vi "test-Mecanum-Odometry-Test1.vi"() -> (3 "All tests passed":bool)   [LabVIEW 2019]
uses:
  <vilib>/Rock Robotics/WPI/ThirdParty/JAS_Junk/TrajLib/Trajectory_Library.lvlib
panel:
  out "Test 4":bool
  out "Test 3":bool
  out "Test 2":bool
  out "Test 1":bool
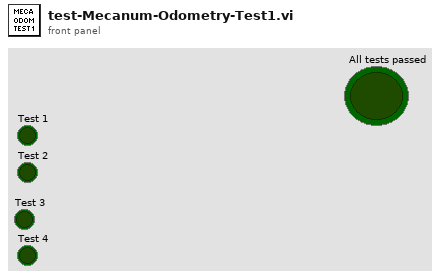
[diagram p1: front panel]
types:
  T1 = typedef "Trajectory_Library.lvlib/ROTATION2D.ctl" = cluster{"VALUE":dbl, "COS":dbl, "SIN":dbl}
  T2 = typedef "Trajectory_Library.lvlib/POSE2D.ctl" = cluster{"TRANSLATION":T3, "ROTATION":T1}
  T3 = typedef "Trajectory_Library.lvlib/TRANSLATION2D.ctl" = cluster{"X":dbl, "Y":dbl}
  T4 = typedef "Trajectory_Library.lvlib/MECA_WHEEL_SPEEDS.ctl" = cluster{"FrontLeftSpeed":dbl, "FrontRightSpeed":dbl, "RearLeftSpeed":dbl, "RearRightSpeed":dbl}
  T5 = typedef "Trajectory_Library.lvlib/MECA_DRIVE_KINEMATICS.ctl" = cluster{"FrontLeft":T3, "FrontRight":T3, "RearLeft":T3, "RearRight":T3, "InverseKinematics":T6, "ForwardKinematics":T6, "PrevCoR":T3}
  T6 = typedef "NI_Matrix.lvlib/RealMatrix.ctl" = dbl[][]
  T7 = typedef "Trajectory_Library.lvlib/MECA_DRIVE_ODOMETRY.ctl" = cluster{"POSE":T2, "PrevTime":dbl, "GyroOffset":T1, "PreviousAngle":T1, "Kinematics":T5}
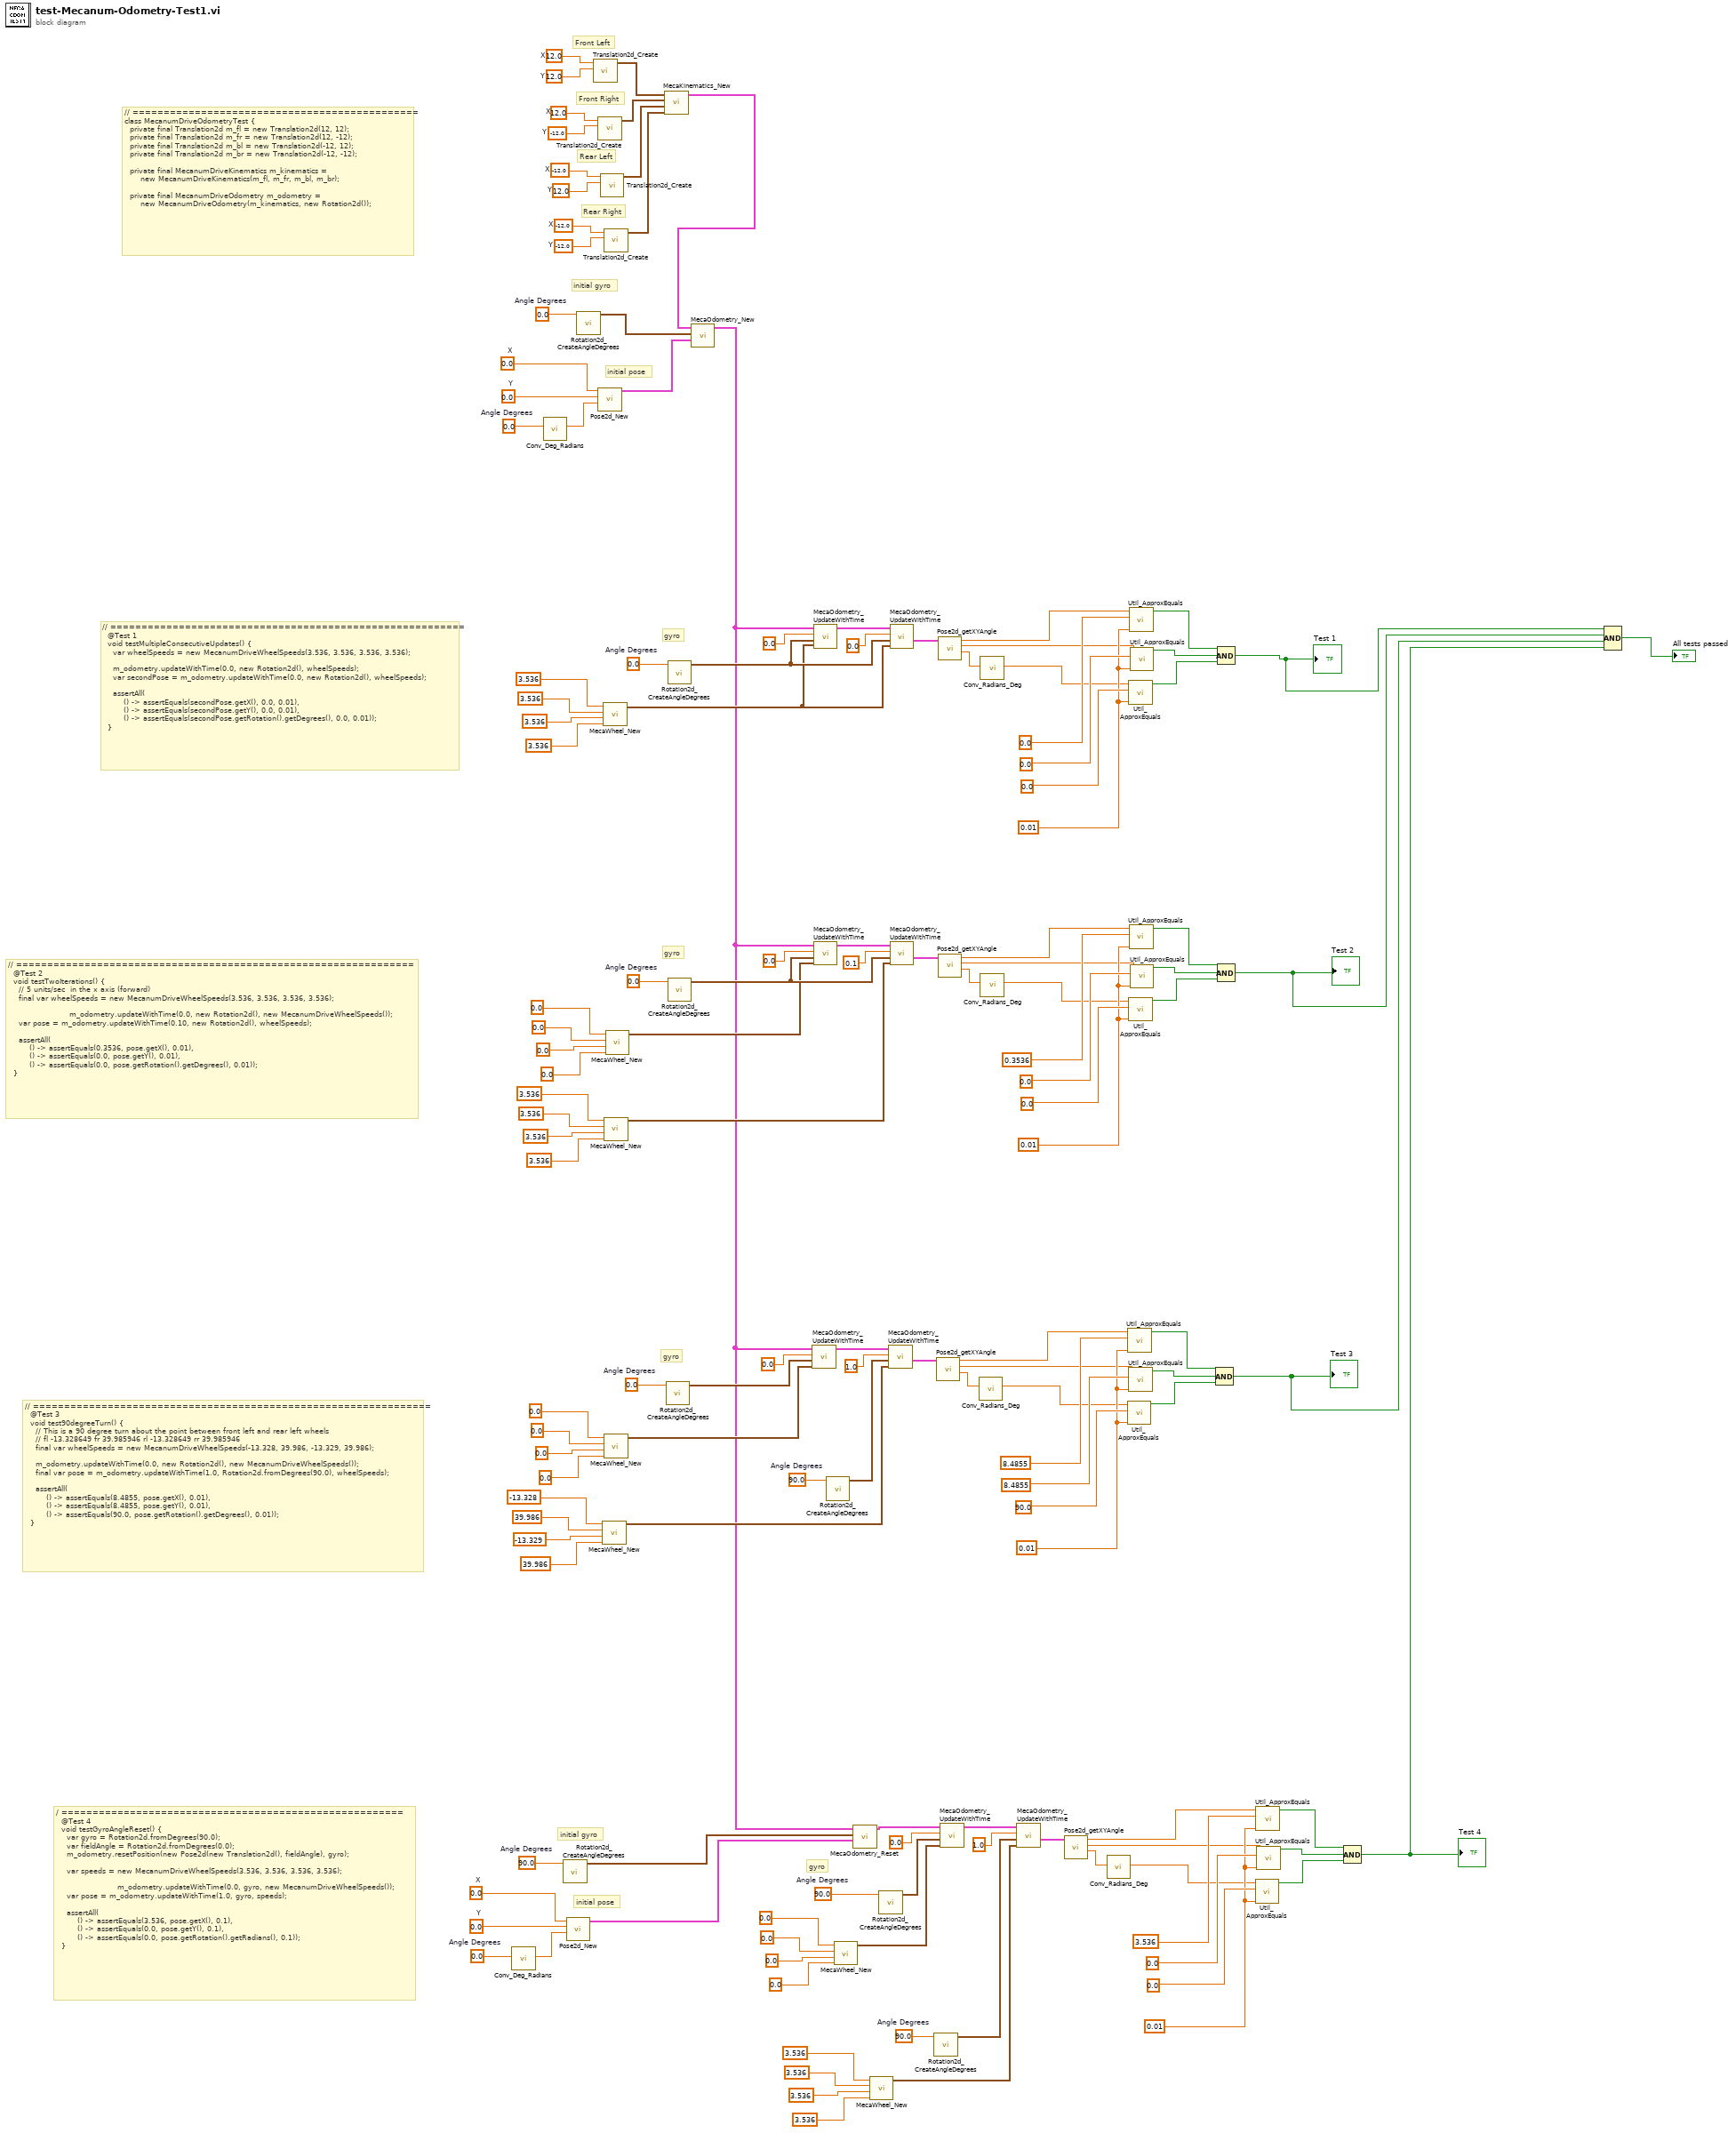
[diagram p0: block diagram]
diagram:
  w6 = 90.0  # Angle Degrees
  w10 = 0.0  # X
  w9 = 0.0  # Y
  w7 = 0.0  # Angle Degrees
  w14 = 90.0  # Angle Degrees
  w28 = 90.0  # Angle Degrees
  w35 = 0.01 ("Tolerance")
  w44 = 90.0  # Angle Degrees
  w58 = 0.0  # Angle Degrees
  w65 = 0.01 ("Tolerance")
  w86 = 0.0  # Angle Degrees
  w93 = 0.01 ("Tolerance")
  w108 = 0.0  # Angle Degrees
  w115 = 0.0  # Angle Degrees
  w120 = 0.0  # X
  w119 = 0.0  # Y
  w117 = 0.0  # Angle Degrees
  w121 = 0.01 ("Tolerance")
  w136 = -12.0  # X
  w135 = -12.0  # Y
  w134 = -12.0  # X
  w133 = 12.0  # Y
  w132 = 12.0  # X
  w131 = -12.0  # Y
  w130 = 12.0  # X
  w129 = 12.0  # Y
  # "initial gyro"
  # "initial pose"
  # "gyro"
  # "/ =======================================================\n  @Test 4\n  void testGyroAngleReset() {\n    var gyro = Rotation2d.fromDegrees(90.0);\n    var fieldAngle = Rotation2d.fromDegrees(0.0);\n    m_odometry.resetPosition(new Pose2d(new Translation2d(), fieldAngle), gyro);\n\n    var speeds = new MecanumDriveWheelSpeeds(3.536, 3.536, 3.536, 3.536);\n\n                       m_odometry.updateWithTime(0.0, gyro, new MecanumDriveWheelSpeeds());\n    var pose = m_odometry.updateWithTime(1.0, gyro, speeds);\n\n    assertAll(\n        () -> assertEquals(3.536, pose.getX(), 0.1),\n        () -> assertEquals(0.0, pose.getY(), 0.1),\n        () -> assertEquals(0.0, pose.getRotation().getRadians(), 0.1));\n  }"
  # "gyro"
  # "// ================================================================\n  @Test 3\n  void test90degreeTurn() {\n    // This is a 90 degree turn about the point between front left and rear left wheels\n    // fl -13.328649 fr 39.985946 rl -13.328649 rr 39.985946\n    final var wheelSpeeds = new MecanumDriveWheelSpeeds(-13.328, 39.986, -13.329, 39.986);\n\n    m_odometry.updateWithTime(0.0, new Rotation2d(), new MecanumDriveWheelSpeeds());\n    final var pose = m_odometry.updateWithTime(1.0, Rotation2d.fromDegrees(90.0), wheelSpeeds);\n\n    assertAll(\n        () -> assertEquals(8.4855, pose.getX(), 0.01),\n        () -> assertEquals(8.4855, pose.getY(), 0.01),\n        () -> assertEquals(90.0, pose.getRotation().getDegrees(), 0.01));\n  }"
  # "gyro"
  # "// ================================================================\n  @Test 2\n  void testTwoIterations() {\n    // 5 units/sec  in the x axis (forward)\n    final var wheelSpeeds = new MecanumDriveWheelSpeeds(3.536, 3.536, 3.536, 3.536);\n\n                       m_odometry.updateWithTime(0.0, new Rotation2d(), new MecanumDriveWheelSpeeds());\n    var pose = m_odometry.updateWithTime(0.10, new Rotation2d(), wheelSpeeds);\n\n    assertAll(\n        () -> assertEquals(0.3536, pose.getX(), 0.01),\n        () -> assertEquals(0.0, pose.getY(), 0.01),\n        () -> assertEquals(0.0, pose.getRotation().getDegrees(), 0.01));\n  }"
  # "gyro"
  # "initial gyro"
  # "initial pose"
  # "// =========================================================\n  @Test 1\n  void testMultipleConsecutiveUpdates() {\n    var wheelSpeeds = new MecanumDriveWheelSpeeds(3.536, 3.536, 3.536, 3.536);\n\n    m_odometry.updateWithTime(0.0, new Rotation2d(), wheelSpeeds);\n    var secondPose = m_odometry.updateWithTime(0.0, new Rotation2d(), wheelSpeeds);\n\n    assertAll(\n        () -> assertEquals(secondPose.getX(), 0.0, 0.01),\n        () -> assertEquals(secondPose.getY(), 0.0, 0.01),\n        () -> assertEquals(secondPose.getRotation().getDegrees(), 0.0, 0.01));\n  }"
  # "Rear Right"
  # "Rear Left"
  # "Front Right"
  # "Front Left"
  # "// ==============================================\nclass MecanumDriveOdometryTest {\n  private final Translation2d m_fl = new Translation2d(12, 12);\n  private final Translation2d m_fr = new Translation2d(12, -12);\n  private final Translation2d m_bl = new Translation2d(-12, 12);\n  private final Translation2d m_br = new Translation2d(-12, -12);\n\n  private final MecanumDriveKinematics m_kinematics =\n      new MecanumDriveKinematics(m_fl, m_fr, m_bl, m_br);\n\n  private final MecanumDriveOdometry m_odometry =\n      new MecanumDriveOdometry(m_kinematics, new Rotation2d());"
  n1 = call <vilib>:"Conv_Deg_Radians.vi"("Degress"=w7) -> ("Radians"=w8:dbl)  [unwired: 10 in]
  n2 = call <vilib>:"Conv_Deg_Radians.vi"("Degress"=w117) -> ("Radians"=w118:dbl)  [unwired: 10 in]
  n3 = call <vilib>:"Rotation2d_CreateAngleDegrees.vi"("Angle_Degrees"=w6) -> ("ROTATION"=w5:T1)  [unwired: 10 in]
  n4 = call <vilib>:"Pose2d_New.vi"("Heading"=w8, "Y"=w9, "X"=w10) -> ("out POSe"=w4:T2)  [unwired: 8 in]
  n5 = call <vilib>:"Rotation2d_CreateAngleDegrees.vi"("Angle_Degrees"=w115) -> ("ROTATION"=w2:T1)  [unwired: 10 in]
  n6 = call <vilib>:"Translation2d_Create.vi"("Y"=w129, "X"=w130) -> ("TRANSLATION"=w137:T3)  [unwired: 9 in]
  n7 = call <vilib>:"Translation2d_Create.vi"("Y"=w131, "X"=w132) -> ("TRANSLATION"=w138:T3)  [unwired: 9 in]
  n8 = call <vilib>:"Pose2d_New.vi"("Heading"=w118, "Y"=w119, "X"=w120) -> ("out POSe"=w116:T2)  [unwired: 8 in]
  n9 = call <vilib>:"Translation2d_Create.vi"("Y"=w133, "X"=w134) -> ("TRANSLATION"=w139:T3)  [unwired: 9 in]
  n10 = call <vilib>:"MecaWheel_New.vi"("RearRightSpeed"=39.986, "RearLeftSpeed"=-13.329, "FrontRightSpeed"=39.986, "FrontLeftSpeed"=-13.328) -> ("MECA_WHEEL_SPEEDS"=w50:T4)  [unwired: 7 in]
  n11 = call <vilib>:"MecaWheel_New.vi"("RearRightSpeed"=3.536, "RearLeftSpeed"=3.536, "FrontRightSpeed"=3.536, "FrontLeftSpeed"=3.536) -> ("MECA_WHEEL_SPEEDS"=w100:T4)  [unwired: 7 in]
  n12 = call <vilib>:"Translation2d_Create.vi"("Y"=w135, "X"=w136) -> ("TRANSLATION"=w140:T3)  [unwired: 9 in]
  n13 = call <vilib>:"MecaWheel_New.vi"("RearRightSpeed"=3.536, "RearLeftSpeed"=3.536, "FrontRightSpeed"=3.536, "FrontLeftSpeed"=3.536) -> ("MECA_WHEEL_SPEEDS"=w78:T4)  [unwired: 7 in]
  n14 = call <vilib>:"MecaWheel_New.vi"("RearRightSpeed"=0.0, "RearLeftSpeed"=0.0, "FrontRightSpeed"=0.0, "FrontLeftSpeed"=0.0) -> ("MECA_WHEEL_SPEEDS"=w45:T4)  [unwired: 7 in]
  n15 = call <vilib>:"MecaWheel_New.vi"("RearRightSpeed"=0.0, "RearLeftSpeed"=0.0, "FrontRightSpeed"=0.0, "FrontLeftSpeed"=0.0) -> ("MECA_WHEEL_SPEEDS"=w73:T4)  [unwired: 7 in]
  n16 = call <vilib>:"MecaKinematics_New.vi"("RearRight"=w140, "RearLeft"=w139, "FrontRight"=w138, "FrontLeft"=w137) -> ("MECA_DRIVE_KINEMATICS"=w1:T5)  [unwired: 7 in]
  n17 = call <vilib>:"Rotation2d_CreateAngleDegrees.vi"("Angle_Degrees"=w58) -> ("ROTATION"=w56:T1)  [unwired: 10 in]
  n18 = call <vilib>:"Rotation2d_CreateAngleDegrees.vi"("Angle_Degrees"=w108) -> ("ROTATION"=w106:T1)  [unwired: 10 in]
  n19 = call <vilib>:"Rotation2d_CreateAngleDegrees.vi"("Angle_Degrees"=w86) -> ("ROTATION"=w84:T1)  [unwired: 10 in]
  n20 = call <vilib>:"MecaOdometry_New.vi"("Initial Pose2d"=w116, "GyroOffset"=w2, "Mecanum Kinematics"=w1) -> ("MECA_DRIVE_ODOMETRY"=w11:T7)  [unwired: 8 in]
  n21 = call <vilib>:"MecaOdometry_UpdateWithTime.vi"("WheelSpeeds"=w45, "GyroAngle"=w56, "CurrentTime"=0.0, "in MECA_DRIVE_ODOMETRY"=w11) -> ("out MECA_DRIVE_ODOMETRY"=w60:T7)  [unwired: 6 in, 1 out]
  n22 = call <vilib>:"MecaOdometry_UpdateWithTime.vi"("WheelSpeeds"=w100, "GyroAngle"=w106, "CurrentTime"=0.0, "in MECA_DRIVE_ODOMETRY"=w11) -> ("out MECA_DRIVE_ODOMETRY"=w110:T7)  [unwired: 6 in, 1 out]
  n23 = call <vilib>:"MecaOdometry_UpdateWithTime.vi"("WheelSpeeds"=w73, "GyroAngle"=w84, "CurrentTime"=0.0, "in MECA_DRIVE_ODOMETRY"=w11) -> ("out MECA_DRIVE_ODOMETRY"=w88:T7)  [unwired: 6 in, 1 out]
  n24 = call <vilib>:"Rotation2d_CreateAngleDegrees.vi"("Angle_Degrees"=w44) -> ("ROTATION"=w43:T1)  [unwired: 10 in]
  n25 = call <vilib>:"MecaWheel_New.vi"("RearRightSpeed"=0.0, "RearLeftSpeed"=0.0, "FrontRightSpeed"=0.0, "FrontLeftSpeed"=0.0) -> ("MECA_WHEEL_SPEEDS"=w15:T4)  [unwired: 7 in]
  n26 = call <vilib>:"MecaOdometry_Reset.vi"("POSE"=w4, "GyroOffset"=w5, "in MECA_DRIVE_ODOMETRY"=w11) -> ("out MECA_DRIVE_ODOMETRY"=w12:T7)  [unwired: 8 in]
  n27 = call <vilib>:"MecaWheel_New.vi"("RearRightSpeed"=3.536, "RearLeftSpeed"=3.536, "FrontRightSpeed"=3.536, "FrontLeftSpeed"=3.536) -> ("MECA_WHEEL_SPEEDS"=w20:T4)  [unwired: 7 in]
  n28 = call <vilib>:"Rotation2d_CreateAngleDegrees.vi"("Angle_Degrees"=w28) -> ("ROTATION"=w26:T1)  [unwired: 10 in]
  n29 = call <vilib>:"MecaOdometry_UpdateWithTime.vi"("WheelSpeeds"=w50, "GyroAngle"=w43, "CurrentTime"=1.0, "in MECA_DRIVE_ODOMETRY"=w60) -> ("POSE"=w55:T2)  [unwired: 6 in, 1 out]
  n30 = call <vilib>:"MecaOdometry_UpdateWithTime.vi"("WheelSpeeds"=w100, "GyroAngle"=w106, "CurrentTime"=0.0, "in MECA_DRIVE_ODOMETRY"=w110) -> ("POSE"=w105:T2)  [unwired: 6 in, 1 out]
  n31 = call <vilib>:"MecaOdometry_UpdateWithTime.vi"("WheelSpeeds"=w78, "GyroAngle"=w84, "CurrentTime"=0.1, "in MECA_DRIVE_ODOMETRY"=w88) -> ("POSE"=w83:T2)  [unwired: 6 in, 1 out]
  n32 = call <vilib>:"Rotation2d_CreateAngleDegrees.vi"("Angle_Degrees"=w14) -> ("ROTATION"=w13:T1)  [unwired: 10 in]
  n33 = call <vilib>:"Pose2d_getXYAngle.vi"("in POSE"=w55) -> ("Angle"=w54:dbl, "Y"=w52:dbl, "X"=w53:dbl)  [unwired: 8 in]
  n34 = call <vilib>:"Pose2d_getXYAngle.vi"("in POSE"=w105) -> ("Angle"=w104:dbl, "Y"=w102:dbl, "X"=w103:dbl)  [unwired: 8 in]
  n35 = call <vilib>:"Pose2d_getXYAngle.vi"("in POSE"=w83) -> ("Angle"=w82:dbl, "Y"=w80:dbl, "X"=w81:dbl)  [unwired: 8 in]
  n36 = call <vilib>:"MecaOdometry_UpdateWithTime.vi"("WheelSpeeds"=w15, "GyroAngle"=w26, "CurrentTime"=0.0, "in MECA_DRIVE_ODOMETRY"=w12) -> ("out MECA_DRIVE_ODOMETRY"=w30:T7)  [unwired: 6 in, 1 out]
  n37 = call <vilib>:"Conv_Radians_Deg.vi"("Radians"=w54) -> ("Degrees"=w51:dbl)  [unwired: 10 in]
  n38 = call <vilib>:"Conv_Radians_Deg.vi"("Radians"=w104) -> ("Degrees"=w101:dbl)  [unwired: 10 in]
  n39 = call <vilib>:"Conv_Radians_Deg.vi"("Radians"=w82) -> ("Degrees"=w79:dbl)  [unwired: 10 in]
  n40 = call <vilib>:"MecaOdometry_UpdateWithTime.vi"("WheelSpeeds"=w20, "GyroAngle"=w13, "CurrentTime"=1.0, "in MECA_DRIVE_ODOMETRY"=w30) -> ("POSE"=w25:T2)  [unwired: 6 in, 1 out]
  n41 = call <vilib>:"Pose2d_getXYAngle.vi"("in POSE"=w25) -> ("Angle"=w24:dbl, "Y"=w22:dbl, "X"=w23:dbl)  [unwired: 8 in]
  n42 = call <vilib>:"Conv_Radians_Deg.vi"("Radians"=w24) -> ("Degrees"=w21:dbl)  [unwired: 10 in]
  n43 = call <vilib>:"Util_ApproxEquals.vi"("Tolerance"=w65, "Value 2"=90.0, "Value 1"=w51) -> ("ApproxEquals"=w66:bool)  [unwired: 8 in]
  n44 = call <vilib>:"Util_ApproxEquals.vi"("Tolerance"=w65, "Value 2"=8.4855, "Value 1"=w53) -> ("ApproxEquals"=w68:bool)  [unwired: 8 in]
  n45 = call <vilib>:"Util_ApproxEquals.vi"("Tolerance"=w121, "Value 2"=0.0, "Value 1"=w101) -> ("ApproxEquals"=w123:bool)  [unwired: 8 in]
  n46 = call <vilib>:"Util_ApproxEquals.vi"("Tolerance"=w93, "Value 2"=0.0, "Value 1"=w79) -> ("ApproxEquals"=w94:bool)  [unwired: 8 in]
  n47 = call <vilib>:"Util_ApproxEquals.vi"("Tolerance"=w65, "Value 2"=8.4855, "Value 1"=w52) -> ("ApproxEquals"=w67:bool)  [unwired: 8 in]
  n48 = call <vilib>:"Util_ApproxEquals.vi"("Tolerance"=w121, "Value 2"=0.0, "Value 1"=w103) -> ("ApproxEquals"=w125:bool)  [unwired: 8 in]
  n49 = call <vilib>:"Util_ApproxEquals.vi"("Tolerance"=w93, "Value 2"=0.3536, "Value 1"=w81) -> ("ApproxEquals"=w96:bool)  [unwired: 8 in]
  n50 = call <vilib>:"Util_ApproxEquals.vi"("Tolerance"=w121, "Value 2"=0.0, "Value 1"=w102) -> ("ApproxEquals"=w124:bool)  [unwired: 8 in]
  n51 = call <vilib>:"Util_ApproxEquals.vi"("Tolerance"=w93, "Value 2"=0.0, "Value 1"=w80) -> ("ApproxEquals"=w95:bool)  [unwired: 8 in]
  n52 = Compound Arithmetic op=AND(w68, w67, w66) -> (w42:bool)
  "Test 3" <- w42
  n53 = Compound Arithmetic op=AND(w125, w124, w123) -> (w122:bool)
  "Test 1" <- w122
  n54 = Compound Arithmetic op=AND(w96, w95, w94) -> (w72:bool)
  "Test 2" <- w72
  n55 = call <vilib>:"Util_ApproxEquals.vi"("Tolerance"=w35, "Value 2"=0.0, "Value 1"=w21) -> ("ApproxEquals"=w36:bool)  [unwired: 8 in]
  n56 = call <vilib>:"Util_ApproxEquals.vi"("Tolerance"=w35, "Value 2"=3.536, "Value 1"=w23) -> ("ApproxEquals"=w38:bool)  [unwired: 8 in]
  n57 = call <vilib>:"Util_ApproxEquals.vi"("Tolerance"=w35, "Value 2"=0.0, "Value 1"=w22) -> ("ApproxEquals"=w37:bool)  [unwired: 8 in]
  n58 = Compound Arithmetic op=AND(w38, w37, w36) -> (w3:bool)
  "Test 4" <- w3
  n59 = Compound Arithmetic op=AND(w122, w72, w42, w3) -> (→"All tests passed":bool)
